vi "Queue Comms FG.vi"(8 "error in":errorcluster, 9 "Action":T1, 11 "queue in":refnum<queue>) -> (0 "error out":errorcluster, 3 "queue out":refnum<queue>)   [LabVIEW 2018, in "LED Control Module.lvlib"]
uses:
  LED Control Module.lvlib
  Private Controls/Queue FG Action.ctl
  Private Controls/Module Data Cluster.ctl
  Private Controls/Module Action.ctl
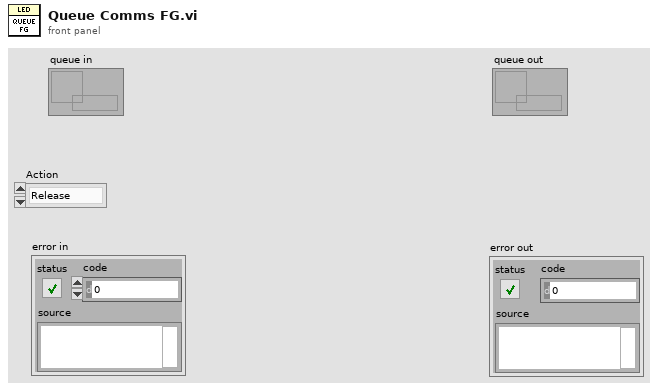
[diagram p1: front panel]
types:
  T1 = typedef "LED Control Module.lvlib/Queue FG Action.ctl" = enum16{"Release", "Get", "Set"}
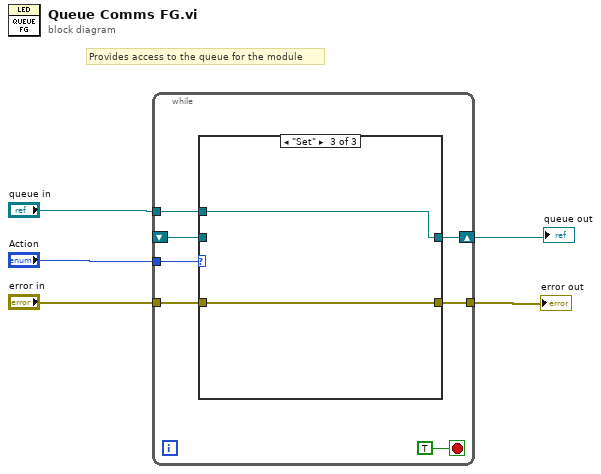
[diagram p0: block diagram]
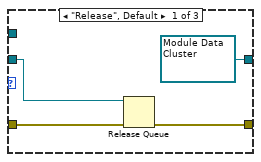
[diagram p2: hidden frame]
diagram:
  # "Provides access to the queue for the module"
  n1 = while {
    tunnel: "Action" -> [w12]
    shift-right: [w9] -> w1
    shift-left: _ -> [w11]
    tunnel: "error in" -> [w10]
    tunnel: "queue in" -> [w8]
    tunnel: [w6] -> w3
    stop <- TRUE stop-if-true
    n2 = case shown="\"Set\"" w12 {
      tunnel: w11 -> [w16 w18 _]
      tunnel: w10 -> [w15 w17 w19]
      tunnel: [refnum<queue> refnum ("queue in") w18 w20] -> w9
      tunnel: w8 -> [_ _ w20]
      tunnel: [w14 w17 w19] -> w6
      frame "Release", Default {
        n3 = Release Queue(queue=w16, error in (no error)=w15) -> (error out=w14:errorcluster)  [unwired: 1 in, 2 out]
      }
      frame "Get" {
      }
      frame "Set" {
      }
    }
  }
  "error out" <- w3
  "queue out" <- w1
